vi "path steer.vi"() -> (0 "path size":i32=100, 3 "handle":dbl=-6.682613607342708)   [LabVIEW 2015]
uses:
  G_ALL.vi
panel:
  out "Array 2":dbl[][](array[numeric])
  out "dist":dbl[](array[numeric])
  in  "Numeric":dbl=2.0 format="%#_13g"
  out "Array":dbl[](array[numeric])=[0.2515789699310972, 0.252650768433432, 0.2537225783523809, 0.25479439920413827, 0.255866230504671, 0.2569380717700824, 0.25800992251627125, 0.2590817822591362, 0.2601536505146442, 0.26122552679873934, 0.2622974106272295, 0.26137675907978064, 0.26006281964444045, 0.25874890404318196, 0.2574350130090579, 0.2561211472750756, 0.25480730757403763, 0.2534934946388148, 0.2521797092019597, 0.25086595199611567, 0.24955222375374433]
  in  "y":dbl=3.0
  out "normal dist":dbl=0.8942045357809025
  out "min value":dbl=0.5
  out "size(s)":i32
  out "map_track":dbl[][](array[numeric])=[[0.15625, -20.718822434390773], [0.2395675475439587, -20.20422919806885], [0.3195188405478051, -19.689494249463262]]
  out "XY Graph":cluster{"Y":dbl[], "Y":dbl[]}[](graph)=[{"Y"=[0.15625, 0.2395675475439587, 0.3195188405478051], "Y"=[-20.718822434390773, -20.20422919806885, -19.689494249463262]}, {"Y"=array[360 elements], "Y"=array[360 elements]}, {"Y"=[0.15625, 0.2395675475439587, 0.3195188405478051], "Y"=[-20.718822434390773, -20.20422919806885, -19.689494249463262]}]
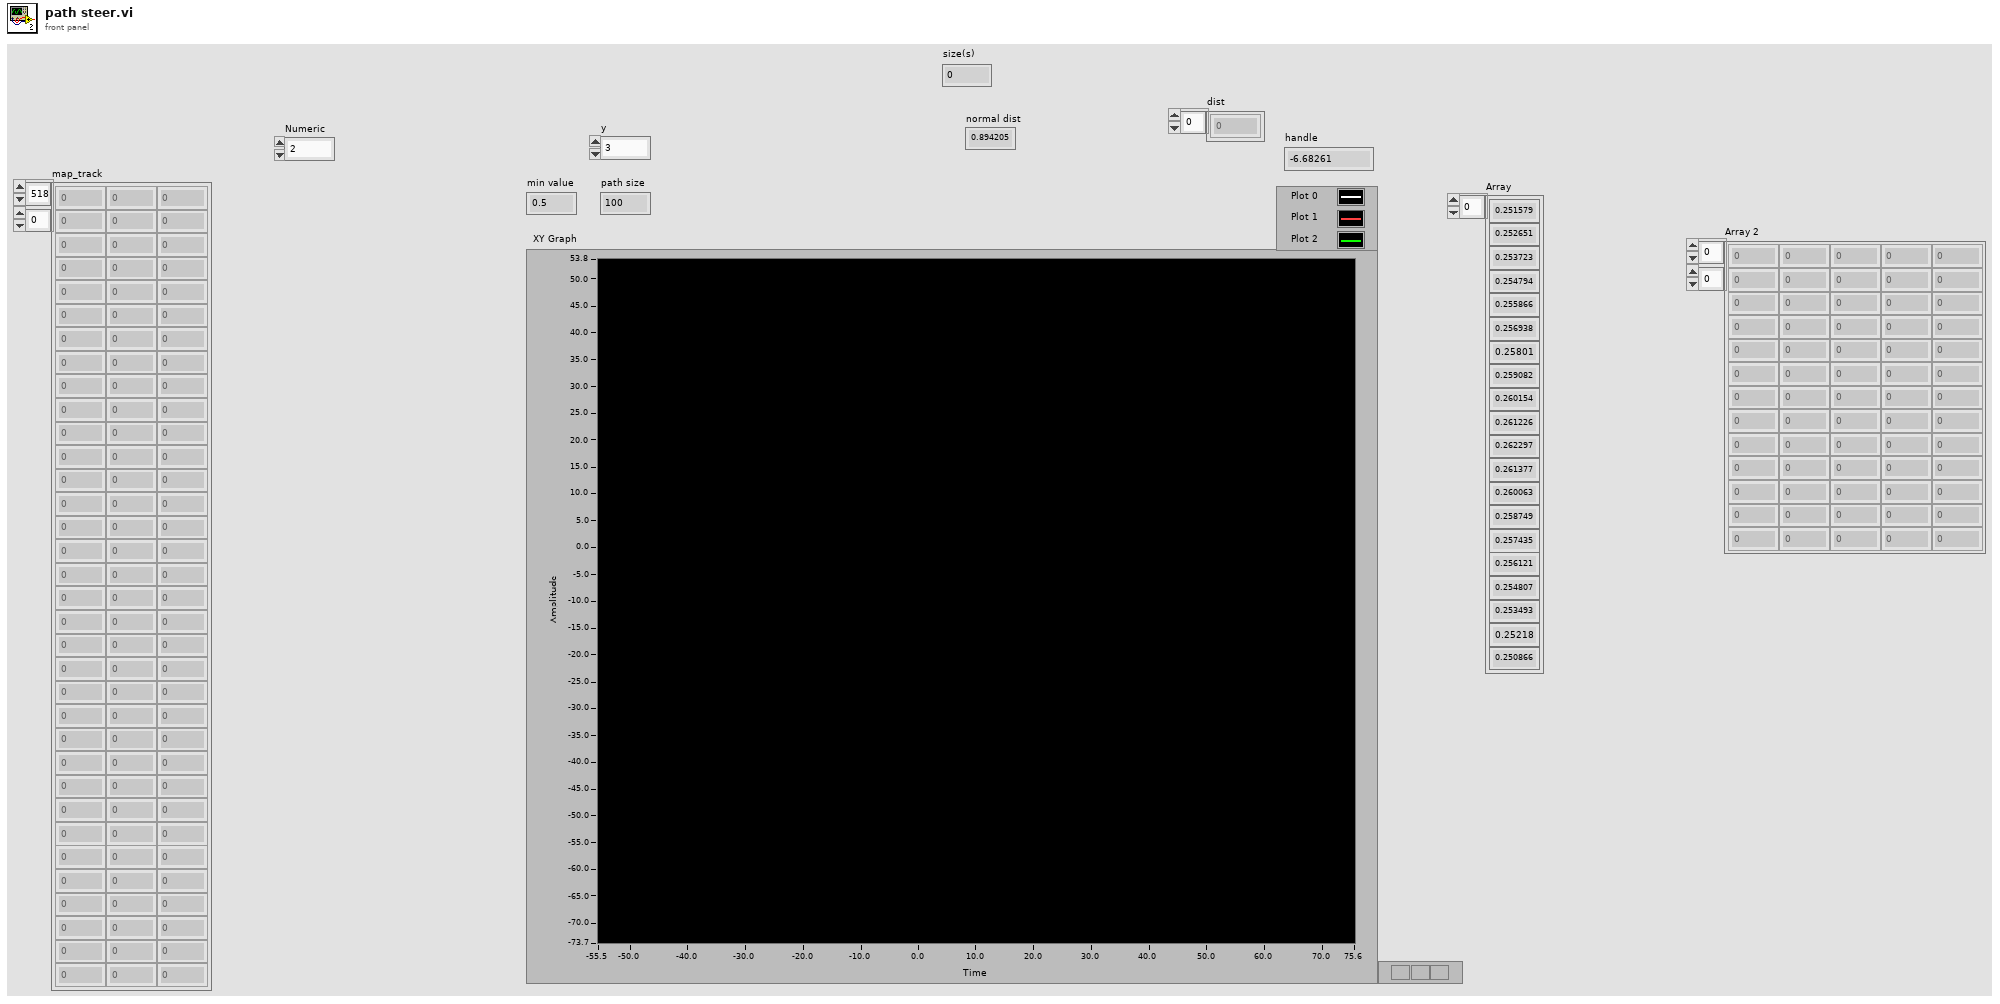
[diagram p1: front panel]
types:
  T1 = cluster{"C_Wheel base":dbl, "ratio_steer":dbl, "Overall width":dbl, "af":dbl, "turn radius":dbl, "eval":dbl, "ap":dbl, "an":dbl, "Vmax":dbl, "mu":dbl, "Vlast":dbl}
  T2 = cluster{"Steer_input":dbl, "Steer_output":dbl, "VS_des":dbl, "VS_can":dbl, "heading":dbl, "auto":bool, "run":bool, "x":dbl, "y":dbl}
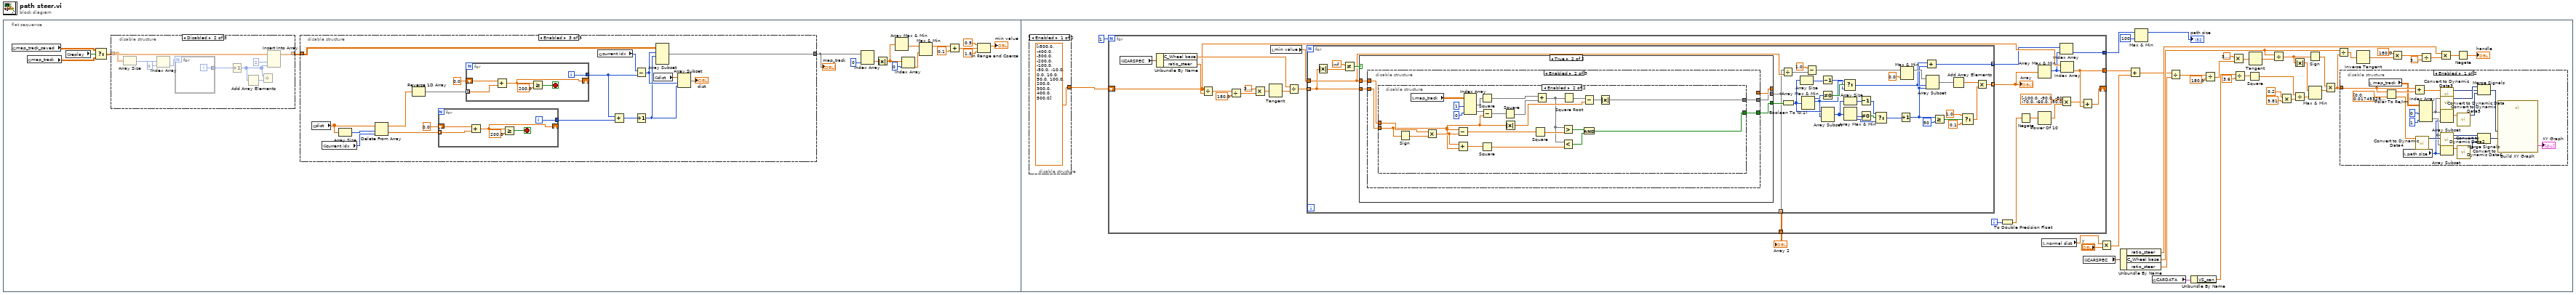
[diagram p0: block diagram]
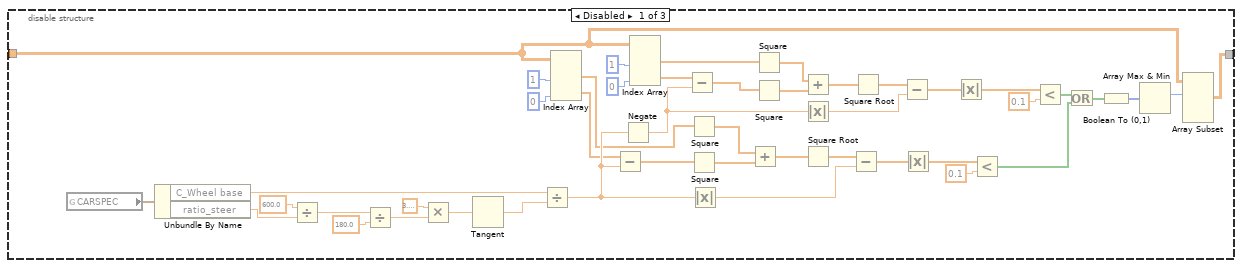
[diagram p2: hidden frame]
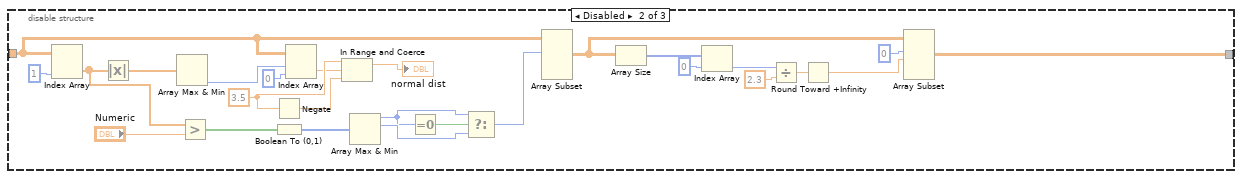
[diagram p3: hidden frame]
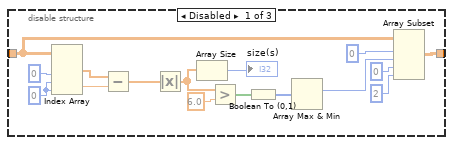
[diagram p4: hidden frame]
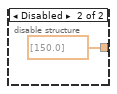
[diagram p6: hidden frame]
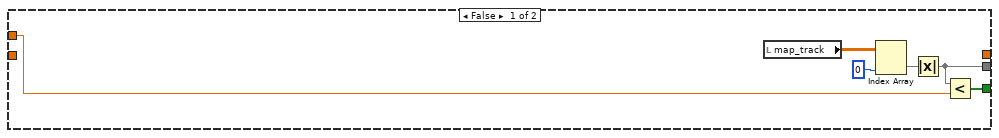
[diagram p8: hidden frame]
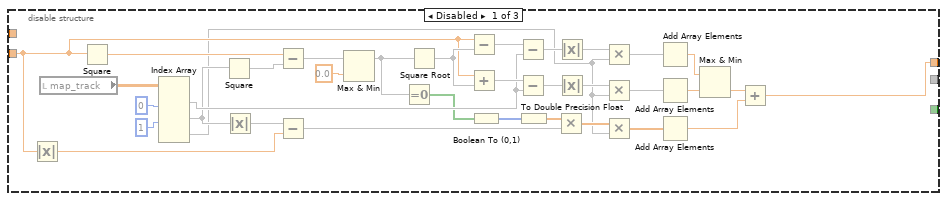
[diagram p9: hidden frame]
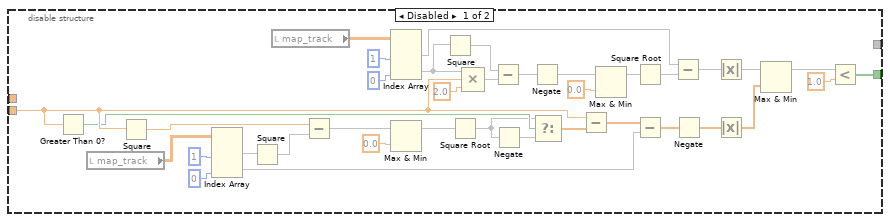
[diagram p10: hidden frame]
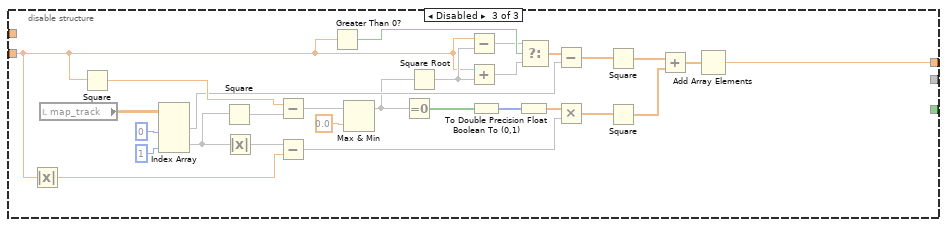
[diagram p11: hidden frame]
diagram:
  n1 = flat-sequence {
    frame #0 {
      n2 = global read "G_ALL.vi" "map_track_saved"() -> (w9:dbl[][])
      n3 = global read "G_ALL.vi" "map_track"() -> (w8:dbl[][])
      n4 = global read "G_ALL.vi" "replay"() -> (w10:bool)
      n5 = Select(t=w9, s=w10, f=w8) -> (s? t:f=w7:dbl[][])
      n6 = disable-structure shown="Disabled" {
        disable-tunnel: w7 -> [w128 w140 w146]
        disable-tunnel: [w123 w138 w146] -> w13
        frame Disabled {
          w133 = 0 ("index (col)")
          n7 = Index Array(array=w128, index (col) #1=0 ("disabled index (col)"), index (row) #2=w133, index (col) #2=w133) -> (element #1=w132:dbl[], element #2=w131:dbl)  [unwired: 1 in]
          n8 = Subtract(x=w132, y=w131) -> (x-y=w130:dbl[])
          n9 = Absolute Value(x=w130) -> (abs(x)=w122:dbl[])
          n10 = Array Size(array=w122) -> (size(s)=→"size(s)":i32)
          n11 = Greater?(x=w122, y=6.0) -> (0:w134:bool[])
          n12 = Boolean To (0,1)(Boolean=w134) -> (0, 1=w129:i16[])
          n13 = Array Max & Min(array=w129) -> (max index (indices)=w127:i32)  [unwired: 3 out]
          n14 = Array Subset(array=w128, index (row)=0 ("index"), length (row)=w127, index (col)=0 ("index"), length (col)=2 ("length")) -> (w123:dbl[][])
        }
        frame Disabled {
          n15 = Array Size(array=w140) -> (size(s)=w144:i32[])
          n16 = Index Array(array=w144, index=0) -> (element=w142:i32)
          n17 = for {
            N: w142 -> [_]
            tunnel: [w145] -> w141 mode=indexing
            i -> [w145]
          }
          n18 = Increment(x=w141) -> (x+1=w136:i32[])
          n19 = Add Array Elements(numeric array=w136) -> (sum=w137:i32)
          n20 = Divide(x=w136, y=w137) -> ()  [unwired: 1 out]
          n21 = Insert Into Array(array=w140, index (col)=2 ("disabled index (col)"), new element=w136) -> (w138:dbl[][])  [unwired: 1 in]
        }
        frame Enabled {
        }
      }
      n22 = disable-structure shown="Enabled" {
        disable-tunnel: w13 -> [w21 w74 w107]
        disable-tunnel: [w19 w87 w106] -> w11
        frame Disabled {
          n23 = global read "G_ALL.vi" "CARSPEC"() -> (w32:T1)
          n24 = Unbundle By Name(w32) -> ("C_Wheel base"=w40:dbl, "ratio_steer"=w38:dbl)
          n25 = Divide(x=600.0, y=w38) -> (x/y=w37:dbl)
          n26 = Divide(x=w37, y=180.0) -> (x/y=w34:dbl)
          n27 = Multiply(x=3.141592653589793, y=w34) -> (x*y=w36:dbl)
          n28 = Tangent(1:w36) -> (0:w39:dbl)
          n29 = Divide(x=w40, y=w39) -> (x/y=w52:dbl)
          n30 = Index Array(array=w21, index (col) #1=1 ("disabled index (col)"), index (col) #2=0 ("disabled index (col)")) -> (element #1=w27:dbl[], element #2=w29:dbl[])  [unwired: 2 in]
          n31 = Subtract(x=w29, y=w52) -> (x-y=w28:dbl[])
          n32 = Negate(x=w52) -> (-x=w53:dbl)
          n33 = Index Array(array=w21, index (col) #1=1 ("disabled index (col)"), index (col) #2=0 ("disabled index (col)")) -> (element #1=w46:dbl[], element #2=w44:dbl[])  [unwired: 2 in]
          n34 = Subtract(x=w44, y=w53) -> (x-y=w45:dbl[])
          n35 = Square(x=w27) -> (x^2=w26:dbl[])
          n36 = Square(x=w28) -> (x^2=w25:dbl[])
          n37 = Absolute Value(x=w52) -> (abs(x)=w24:dbl)
          n38 = Add(x=w26, y=w25) -> (x+y=w22:dbl[])
          n39 = Square(x=w46) -> (x^2=w47:dbl[])
          n40 = Square(x=w45) -> (x^2=w48:dbl[])
          n41 = Add(x=w47, y=w48) -> (x+y=w51:dbl[])
          n42 = Absolute Value(x=w53) -> (abs(x)=w49:dbl)
          n43 = Square Root(x=w22) -> (sqrt(x)=w23:dbl[])
          n44 = Subtract(x=w23, y=w24) -> (x-y=w60:dbl[])
          n45 = Square Root(x=w51) -> (sqrt(x)=w50:dbl[])
          n46 = Subtract(x=w50, y=w49) -> (x-y=w56:dbl[])
          n47 = Absolute Value(x=w60) -> (abs(x)=w62:dbl[])
          n48 = Absolute Value(x=w56) -> (abs(x)=w57:dbl[])
          n49 = Less?(x=w62, y=0.1) -> (x < y?=w63:bool[])
          n50 = Less?(x=w57, y=0.1) -> (x < y?=w59:bool[])
          n51 = Or(x=w59, y=w63) -> (x .or. y?=w54:bool[])
          n52 = Boolean To (0,1)(Boolean=w54) -> (0, 1=w55:i16[])
          n53 = Array Max & Min(array=w55) -> (max index (indices)=w20:i32)  [unwired: 3 out]
          n54 = Array Subset(array=w21, index (row)=w20) -> (w19:dbl[][])  [unwired: 3 in]
        }
        frame Disabled {
          w69 = 3.5 ("upper limit")
          n55 = Index Array(array=w74, index (col)=1 ("disabled index (col)")) -> (element=w76:dbl[])  [unwired: 1 in]
          n56 = Absolute Value(x=w76) -> (abs(x)=w75:dbl[])
          n57 = Array Max & Min(array=w75) -> (min index (indices)=w73:i32)  [unwired: 3 out]
          n58 = Greater?(x=w76, y="Numeric") -> (0:w83:bool[])
          n59 = Negate(x=w69) -> (-x=w70:dbl)
          n60 = Boolean To (0,1)(Boolean=w83) -> (0, 1=w82:i16[])
          n61 = Index Array(array=w74, index (row)=w73, index (col)=0 ("min index(es)")) -> (element=w68:dbl)
          n62 = In Range and Coerce(upper limit=w69, x=w68, lower limit=w70) -> (coerced(x)=→"normal dist":dbl)  [unwired: 1 out]
          n63 = Array Max & Min(array=w82) -> (max value=w79:i16, max index (indices)=w80:i32)  [unwired: 2 out]
          n64 = Equal To 0?(x=w79) -> (x = 0?=w81:bool)
          n65 = Select(t=w79, s=w81, f=w80) -> (s? t:f=w78:i32)
          n66 = Array Subset(array=w74, index (row)=w78) -> (w77:dbl[][])  [unwired: 3 in]
          n67 = Array Size(array=w77) -> (size(s)=w89:i32[])
          n68 = Index Array(array=w89, index=0) -> (element=w67:i32)
          n69 = Divide(x=w67, y=2.3) -> (x/y=w65:dbl)
          n70 = Round Toward +Infinity(x=w65) -> (ceil(x): smallest int >= x=w64:dbl)
          n71 = Array Subset(array=w77, index (row)=0 ("index"), length (row)=w64) -> (w87:dbl[][])  [unwired: 2 in]
        }
        frame Enabled {
          n72 = global read "G_ALL.vi" "dist"() -> (w104:dbl[])
          n73 = global read "G_ALL.vi" "current idx"() -> (w105:i32)
          n74 = Array Size(array=w104) -> (size(s)=w103:i32)
          n75 = Delete From Array(array=w104, length=w103, index=w105) -> (deleted portion=w99:dbl[], array with subset deleted=w102:dbl[])
          n76 = Reverse 1D Array(array=w102) -> (reversed array=w101:dbl[])
          n77 = for {
            tunnel: w99 -> [w112] mode=indexing
            shift-right: [w111] -> _
            shift-left: 0.0 -> [w113]
            tunnel: [w108] -> w95
            i -> [w108]
            stop <- w109 stop-if-true
            n78 = Add(x=w113, y=w112) -> (x+y=w111:dbl)
            n79 = Greater Or Equal?(x=w111, y=200.0) -> (x >= y?=w109:bool)
          }
          n80 = for {
            tunnel: w101 -> [w118] mode=indexing
            shift-right: [w117] -> _
            shift-left: 0.0 -> [w119]
            tunnel: [w114] -> w96
            i -> [w114]
            stop <- w115 stop-if-true
            n81 = Add(x=w119, y=w118) -> (x+y=w117:dbl)
            n82 = Greater Or Equal?(x=w117, y=200.0) -> (x >= y?=w115:bool)
          }
          n83 = global read "G_ALL.vi" "current idx"() -> (w97:i32)
          n84 = Add(x=w96, y=w95) -> (x+y=w94:i32)
          n85 = Subtract(x=w97, y=w96) -> (x-y=w92:i32)
          n86 = Increment(x=w94) -> (x+1=w91:i32)
          n87 = global read "G_ALL.vi" "dist"() -> (w93:dbl[])
          n88 = Array Subset(array=w107, index (row)=w92, length (row)=w91) -> (w106:dbl[][])  [unwired: 2 in]
          n89 = Array Subset(array=w93, index=w92, length=w91) -> (→"dist":dbl[])
        }
      }
      "map_track" <- w11
      n90 = Index Array(array=w11, index (col)=0 ("disabled index (col)")) -> (element=w6:dbl[])  [unwired: 1 in]
      n91 = Absolute Value(x=w6) -> (abs(x)=w17:dbl[])
      n92 = Array Max & Min(array=w17) -> (min value=w14:dbl)  [unwired: 3 out]
      n93 = Index Array(array=w17, index=0) -> (element=w15:dbl)
      n94 = Max & Min(x=w14, y=w15) -> (max(x,y)=w5:dbl)  [unwired: 1 out]
      n95 = Add(x=w5, y=0.1) -> (x+y=w4:dbl)
      n96 = In Range and Coerce(upper limit=0.5, x=w4, lower limit=1.5) -> (coerced(x)=→"min value":dbl)  [unwired: 1 out]
    }
    frame #1 {
      n97 = disable-structure shown="Enabled" {
        disable-tunnel: [dbl[] [-500.0, -400.0, -300.0, -200.0, -100.0, -50.0, -10.0, 0.0, 10.0, 50.0, 100.0, 200.0, 300.0, 400.0, 500.0] ("theta") dbl[] [150.0] ("theta")] -> w148
        frame Enabled {
        }
        frame Disabled {
        }
      }
      n98 = for {
        N: 1 -> [_]
        tunnel: [w221] -> w150
        shift-right: [w222] -> _
        shift-left: w148 -> [w223]
        tunnel: [w215] -> w158
        tunnel: [w214] -> w147
        i -> [w228]
        n99 = global read "G_ALL.vi" "CARSPEC"() -> (w230:T1)
        n100 = Unbundle By Name(w230) -> ("C_Wheel base"=w238:dbl, "ratio_steer"=w236:dbl)
        n101 = Divide(x=w223, y=w236) -> (x/y=w235:dbl[])
        n102 = Divide(x=w235, y=180.0) -> (x/y=w232:dbl[])
        n103 = Multiply(x=3.141592653589793, y=w232) -> (x*y=w234:dbl[])
        n104 = Tangent(1:w234) -> (0:w237:dbl[])
        n105 = local read "min value"() -> (w218:dbl)
        n106 = Divide(x=w238, y=w237) -> (x/y=w229:dbl[])
        n107 = for {
          tunnel: w229 -> [w274] mode=indexing
          tunnel: [w240] -> w219 mode=indexing
          tunnel: w218 -> [w251]
          tunnel: [w248] -> w217 mode=indexing
          tunnel: [w239] -> w214 mode=indexing
          n108 = Absolute Value(x=w274) -> (abs(x)=w272:dbl)
          n109 = Not Equal?(x=inf, y=w272) -> (x != y?=w271:bool)
          n110 = case shown="True" w271 {
            tunnel: [_ w284] -> _
            tunnel: w274 -> [_ w285]
            tunnel: [w278 w283] -> w270
            tunnel: w251 -> [w277 w282]
            tunnel: [w276 w281] -> w239
            frame False {
              n111 = local read "map_track"() -> (w275:dbl[][])
              n112 = Index Array(array=w275, index (col)=0) -> (element=w279:dbl[])  [unwired: 1 in]
              n113 = Absolute Value(x=w279) -> (abs(x)=w276:dbl[])
              n114 = Less?(x=w276, y=w277) -> (x < y?=w278:bool[])
            }
            frame True {
              n115 = disable-structure shown="Enabled" {
                disable-tunnel: w285 -> [w304 w323 w397]
                disable-tunnel: [w295 _ w399] -> w284
                disable-tunnel: [_ w322 _] -> w283
                disable-tunnel: w282 -> [_ w321 _]
                disable-tunnel: [_ w320 _] -> w281
                frame Disabled {
                  n116 = Absolute Value(x=w304) -> (abs(x)=w303:dbl)
                  n117 = local read "map_track"() -> (w293:dbl[][])
                  n118 = Square(x=w304) -> (x^2=w317:dbl)
                  n119 = Index Array(array=w293, index (col) #1=0 ("disabled index (col)"), index (col) #2=1 ("disabled index (col)")) -> (element #1=w306:dbl[], element #2=w298:dbl[], element #3=w286:dbl[])  [unwired: 4 in]
                  n120 = Square(x=w298) -> (x^2=w318:dbl[])
                  n121 = Absolute Value(x=w298) -> (abs(x)=w297:dbl[])
                  n122 = Subtract(x=w317, y=w318) -> (x-y=w309:dbl[])
                  n123 = Subtract(x=w297, y=w303) -> (x-y=w299:dbl[])
                  n124 = Max & Min(x=w309, y=0.0) -> (max(x,y)=w305:dbl[])  [unwired: 1 out]
                  n125 = Equal To 0?(x=w305) -> (x = 0?=w302:bool[])
                  n126 = Square Root(x=w305) -> (sqrt(x)=w316:dbl[])
                  n127 = Subtract(x=w304, y=w316) -> (x-y=w315:dbl[])
                  n128 = Add(x=w304, y=w316) -> (x+y=w314:dbl[])
                  n129 = Boolean To (0,1)(Boolean=w302) -> (0, 1=w301:i16[])
                  n130 = Subtract(x=w315, y=w306) -> (x-y=w313:dbl[])
                  n131 = Subtract(x=w314, y=w306) -> (x-y=w312:dbl[])
                  n132 = To Double Precision Float(number=w301) -> (double precision float=w300:dbl[])
                  n133 = Multiply(x=w300, y=w299) -> (x*y=w292:dbl[])
                  n134 = Absolute Value(x=w313) -> (abs(x)=w290:dbl[])
                  n135 = Absolute Value(x=w312) -> (abs(x)=w288:dbl[])
                  n136 = Multiply(x=w290, y=w286) -> (x*y=w289:dbl[])
                  n137 = Multiply(x=w288, y=w286) -> (x*y=w287:dbl[])
                  n138 = Multiply(x=w292, y=w286) -> (x*y=w291:dbl[])
                  n139 = Add Array Elements(numeric array=w289) -> (sum=w311:dbl)
                  n140 = Add Array Elements(numeric array=w287) -> (sum=w310:dbl)
                  n141 = Add Array Elements(numeric array=w291) -> (sum=w294:dbl)
                  n142 = Max & Min(x=w311, y=w310) -> (min(x,y)=w296:dbl)  [unwired: 1 out]
                  n143 = Add(x=w296, y=w294) -> (x+y=w295:dbl)
                }
                frame Enabled {
                  n144 = disable-structure shown="Enabled" {
                    disable-tunnel: w323 -> [w346 w366]
                    disable-tunnel: [w324 w372] -> w322
                    disable-tunnel: w321 -> [_ w367]
                    disable-tunnel: [_ w362] -> w320
                    frame Disabled {
                      n145 = Greater Than 0?(x=w346) -> (x > 0?=w345:bool)
                      n146 = local read "map_track"() -> (w350:dbl[][])
                      n147 = Square(x=w346) -> (x^2=w349:dbl)
                      n148 = Index Array(array=w350, index (col) #1=1 ("disabled index (col)"), index (col) #2=0 ("index (col)")) -> (element #1=w348:dbl[], element #2=w332:dbl[])  [unwired: 2 in]
                      n149 = Square(x=w348) -> (x^2=w347:dbl[])
                      n150 = local read "map_track"() -> (w359:dbl[][])
                      n151 = Subtract(x=w349, y=w347) -> (x-y=w337:dbl[])
                      n152 = Index Array(array=w359, index (col) #1=1 ("disabled index (col)"), index (col) #2=0 ("disabled index (col)")) -> (element #1=w353:dbl[], element #2=w357:dbl[])  [unwired: 2 in]
                      n153 = Max & Min(x=w337, y=0.0 ("value")) -> (max(x,y)=w336:dbl[])  [unwired: 1 out]
                      n154 = Square(x=w357) -> (x^2=w358:dbl[])
                      n155 = Square Root(x=w336) -> (sqrt(x)=w341:dbl[])
                      n156 = Compound Arithmetic op=MULTIPLY(w357, w346, 2.0 ("value")) -> (w355:dbl[])
                      n157 = Subtract(x=w358, y=w355) -> (x-y=w352:dbl[])
                      n158 = Negate(x=w341) -> (-x=w344:dbl[])
                      n159 = Negate(x=w352) -> (-x=w335:dbl[])
                      n160 = Select(t=w341, s=w345, f=w344) -> (s? t:f=w342:dbl[])
                      n161 = Subtract(x=w346, y=w342) -> (x-y=w334:dbl[])
                      n162 = Max & Min(x=w335, y=0.0 ("value")) -> (max(x,y)=w340:dbl[])  [unwired: 1 out]
                      n163 = Square Root(x=w340) -> (sqrt(x)=w343:dbl[])
                      n164 = Subtract(x=w334, y=w332) -> (x-y=w331:dbl[])
                      n165 = Subtract(x=w353, y=w343) -> (x-y=w330:dbl[])
                      n166 = Negate(x=w331) -> (-x=w329:dbl[])
                      n167 = Absolute Value(x=w330) -> (abs(x)=w328:dbl[])
                      n168 = Absolute Value(x=w329) -> (abs(x)=w327:dbl[])
                      n169 = Max & Min(x=w328, y=w327) -> (max(x,y)=w326:dbl[])  [unwired: 1 out]
                      n170 = Less?(x=w326, y=1.0) -> (x < y?=w324:bool[])
                    }
                    frame Enabled {
                      n171 = Sign(1:w366) -> (0:w371:dbl)
                      n172 = local read "map_track"() -> (w382:dbl[][])
                      n173 = Multiply(x=w367, y=w371) -> (x*y=w370:dbl)
                      n174 = Subtract(x=w366, y=w370) -> (x-y=w369:dbl)
                      n175 = Add(x=w370, y=w366) -> (x+y=w368:dbl)
                      n176 = Index Array(array=w382, index (col) #1=1 ("disabled index (col)"), index (col) #2=0 ("disabled index (col)")) -> (element #1=w379:dbl[], element #2=w381:dbl[])  [unwired: 2 in]
                      n177 = Square(x=w379) -> (x^2=w378:dbl[])
                      n178 = Square(x=w368) -> (x^2=w374:dbl)
                      n179 = Subtract(x=w381, y=w366) -> (x-y=w380:dbl[])
                      n180 = Square(x=w380) -> (x^2=w377:dbl[])
                      n181 = Absolute Value(x=w366) -> (abs(x)=w365:dbl)
                      n182 = Square(x=w369) -> (x^2=w376:dbl)
                      n183 = Add(x=w378, y=w377) -> (x+y=w361:dbl[])
                      n184 = Greater?(x=w361, y=w376) -> (0:w375:bool[])
                      n185 = Less?(x=w361, y=w374) -> (x < y?=w373:bool[])
                      n186 = Square Root(x=w361) -> (sqrt(x)=w364:dbl[])
                      n187 = Subtract(x=w364, y=w365) -> (x-y=w363:dbl[])
                      n188 = And(x=w375, y=w373) -> (x .and. y?=w372:bool[])
                      n189 = Absolute Value(x=w363) -> (abs(x)=w362:dbl[])
                    }
                  }
                }
                frame Disabled {
                  n190 = Absolute Value(x=w397) -> (abs(x)=w395:dbl)
                  n191 = local read "map_track"() -> (w385:dbl[][])
                  n192 = Square(x=w397) -> (x^2=w410:dbl)
                  n193 = Index Array(array=w385, index (col) #1=0 ("disabled index (col)"), index (col) #2=1 ("disabled index (col)")) -> (element #1=w405:dbl[], element #2=w398:dbl[])  [unwired: 2 in]
                  n194 = Square(x=w398) -> (x^2=w411:dbl[])
                  n195 = Absolute Value(x=w398) -> (abs(x)=w396:dbl[])
                  n196 = Subtract(x=w410, y=w411) -> (x-y=w408:dbl[])
                  n197 = Subtract(x=w396, y=w395) -> (x-y=w387:dbl[])
                  n198 = Greater Than 0?(x=w397) -> (x > 0?=w404:bool)
                  n199 = Max & Min(x=w408, y=0.0) -> (max(x,y)=w391:dbl[])  [unwired: 1 out]
                  n200 = Equal To 0?(x=w391) -> (x = 0?=w390:bool[])
                  n201 = Square Root(x=w391) -> (sqrt(x)=w409:dbl[])
                  n202 = Subtract(x=w397, y=w409) -> (x-y=w403:dbl[])
                  n203 = Add(x=w397, y=w409) -> (x+y=w401:dbl[])
                  n204 = Boolean To (0,1)(Boolean=w390) -> (0, 1=w389:i16[])
                  n205 = To Double Precision Float(number=w389) -> (double precision float=w388:dbl[])
                  n206 = Select(t=w403, s=w404, f=w401) -> (s? t:f=w402:dbl[])
                  n207 = Subtract(x=w402, y=w405) -> (x-y=w400:dbl[])
                  n208 = Multiply(x=w388, y=w387) -> (x*y=w386:dbl[])
                  n209 = Square(x=w400) -> (x^2=w394:dbl[])
                  n210 = Square(x=w386) -> (x^2=w393:dbl[])
                  n211 = Add(x=w394, y=w393) -> (x+y=w392:dbl[])
                  n212 = Add Array Elements(numeric array=w392) -> (sum=w399:dbl)
                }
              }
            }
          }
          n213 = Divide(x=w239, y=w251) -> (x/y=w252:dbl[])
          n214 = Boolean To (0,1)(Boolean=w270) -> (0, 1=w262:i16[])
          n215 = Array Size(array=w262) -> (size(s)=w261:i32)
          n216 = Array Max & Min(array=w262) -> (max value=w269:i16, max index (indices)=w259:i32)  [unwired: 2 out]
          n217 = Subtract(x=1.0, y=w252) -> (x-y=w254:dbl[])
          n218 = Decrement(x=w261) -> (x-1=w258:i32)
          n219 = Not Equal To 0?(x=w269) -> (x != 0?=w260:bool)
          n220 = Array Subset(array=w262, index=w259) -> (w267:i16[])  [unwired: 1 in]
          n221 = Select(t=w259, s=w260, f=w258) -> (s? t:f=w249:i32)
          n222 = Array Size(array=w267) -> (size(s)=w266:i32)
          n223 = Array Max & Min(array=w267) -> (min value=w268:i16, min index (indices)=w263:i32)  [unwired: 2 out]
          n224 = Decrement(x=w266) -> (x-1=w264:i32)
          n225 = Not Equal To 0?(x=w268) -> (x != 0?=w265:bool)
          n226 = Select(t=w264, s=w265, f=w263) -> (s? t:f=w257:i32)
          n227 = Increment(x=w257) -> (x+1=w247:i32)
          n228 = Max & Min(x=w254, y=0.0) -> (max(x,y)=w250:dbl[])  [unwired: 1 out]
          n229 = Add(x=w249, y=w247) -> (x+y=w248:i32)
          n230 = Array Subset(array=w250, index=w249, length=w247) -> (w256:dbl[])
          n231 = Greater Or Equal?(x=w247, y=50) -> (x >= y?=w245:bool)
          n232 = Add Array Elements(numeric array=w256) -> (sum=w242:dbl)
          n233 = Select(t=1.0, s=w245, f=0.1) -> (s? t:f=w241:dbl)
          n234 = Multiply(x=w242, y=w241) -> (x*y=w240:dbl)
        }
        "Array" <- w219
        n235 = To Double Precision Float(number=w228) -> (double precision float=w226:dbl)
        n236 = Negate(x=w226) -> (-x=w225:dbl)
        n237 = Array Max & Min(array=w219) -> (max index (indices)=w216:i32)  [unwired: 3 out]
        n238 = Power Of 10(x=w225) -> (10^x=w224:dbl)
        n239 = Index Array(array=w217, index=w216) -> (element=w215:i32)
        n240 = Multiply(x=dbl[] [-100.0, -90.0, -80.0, -70.0, -60.0, -50.0, -40.0, -30.0, -20.0, -10.0, 0.0, 10.0, 20.0, 30.0, 40.0, 50.0, 60.0, 70.0, 80.0, 90.0, 100.0], y=w224) -> (x*y=w220:dbl[])
        n241 = Index Array(array=w223, index=w216) -> (element=w221:dbl)
        n242 = Add(x=w220, y=w221) -> (x+y=w222:dbl[])
      }
      "Array 2" <- w147
      n243 = local read "normal dist"() -> (w155:dbl)
      n244 = global read "G_ALL.vi" "CARSPEC"() -> (w162:T1)
      n245 = Multiply(x=w155, y="y") -> (x*y=w153:dbl)
      n246 = Unbundle By Name(w162) -> ("ratio_steer"=w160:dbl, "C_Wheel base"=w161:dbl, "ratio_steer"=w168:dbl)
      n247 = Add(x=w150, y=w153) -> (x+y=w149:dbl)
      n248 = Max & Min(x=w158, y=100) -> (max(x,y)=→"path size":i32)  [unwired: 1 out]
      n249 = global read "G_ALL.vi" "CARDATA"() -> (w187:T2)
      n250 = Divide(x=w149, y=w168) -> (x/y=w167:dbl)
      n251 = Unbundle By Name(w187) -> ("VS_can"=w170:dbl)
      n252 = Divide(x=w167, y=180.0) -> (x/y=w164:dbl)
      n253 = Multiply(x=3.141592653589793, y=w164) -> (x*y=w166:dbl)
      n254 = Divide(x=w170, y=3.6) -> (x/y=w174:dbl)
      n255 = Square(x=w174) -> (x^2=w175:dbl)
      n256 = Tangent(1:w166) -> (0:w169:dbl)
      n257 = Divide(x=w161, y=w169) -> (x/y=w151:dbl)
      n258 = Multiply(x=0.2, y=9.81) -> (x*y=w176:dbl)
      n259 = Absolute Value(x=w151) -> (abs(x)=w177:dbl)
      n260 = Divide(x=w175, y=w176) -> (x/y=w178:dbl)
      n261 = Sign(1:w151) -> (0:w180:dbl)
      n262 = Max & Min(x=w177, y=w178) -> (max(x,y)=w179:dbl)  [unwired: 1 out]
      n263 = Multiply(x=w180, y=w179) -> (x*y=w188:dbl)
      n264 = Divide(x=w161, y=w188) -> (x/y=w186:dbl)
      n265 = disable-structure shown="Enabled" {
        disable-tunnel: w188 -> [w202 _]
        frame Enabled {
          n266 = local read "map_track"() -> (w199:dbl[][])
          n267 = Polar To Re/Im(2:dbl[] [0.0, 0.017453292519943295, 0.03490658503988659, 0.05235987755982988, 0.06981317007977318, 0.08726646259971647, 0.10471975511965977, 0.12217304763960307, 0.13962634015954636, 0.15707963267948966, 0.17453292519943295, 0.19198621771937624, 0.20943951023931953, 0.22689280275926282, 0.24434609527920614, 0.2617993877991494, 0.2792526803190927, 0.296705972839036, 0.3141592653589793, 0.33161255787892263, 0.3490658503988659, 0.3665191429188092, 0.3839724354387525, 0.40142572795869574, 0.41887902047863906, 0.4363323129985824, 0.45378560551852565, 0.47123889803846897, 0.4886921905584123, 0.5061454830783556, 0.5235987755982988, 0.5410520681182421, 0.5585053606381855, 0.5759586531581287, 0.593411945678072, 0.6108652381980153, 0.6283185307179586, 0.6457718232379019, 0.6632251157578453, 0.6806784082777886, 0.6981317007977318, 0.7155849933176751, 0.7330382858376184, 0.7504915783575618, 0.767944870877505, 0.7853981633974483, 0.8028514559173915, 0.8203047484373349, 0.8377580409572781, 0.8552113334772213, 0.8726646259971648, 0.890117918517108, 0.9075712110370513, 0.9250245035569946, 0.9424777960769379, 0.9599310885968813, 0.9773843811168246, 0.9948376736367678, 1.0122909661567112, 1.0297442586766543, 1.0471975511965976, 1.064650843716541, 1.0821041362364843, 1.0995574287564276, 1.117010721276371, 1.1344640137963142, 1.1519173063162573, 1.1693705988362009, 1.186823891356144, 1.2042771838760875, 1.2217304763960306, 1.239183768915974, 1.2566370614359172, 1.2740903539558606, 1.2915436464758039, 1.3089969389957472, 1.3264502315156905, 1.3439035240356336, 1.3613568165555772, 1.3788101090755203, 1.3962634015954636, 1.413716694115407, 1.4311699866353502, 1.4486232791552935, 1.4660765716752369, 1.48352986419518, 1.5009831567151235, 1.5184364492350666, 1.53588974175501, 1.5533430342749532, 1.5707963267948966, 1.5882496193148399, 1.605702911834783, 1.6231562043547265, 1.6406094968746698, 1.6580627893946132, 1.6755160819145563, 1.6929693744344996, 1.7104226669544427, 1.7278759594743864, 1.7453292519943295, 1.7627825445142729, 1.780235837034216, 1.7976891295541593, 1.8151424220741026, 1.8325957145940461, 1.8500490071139892, 1.8675022996339325, 1.8849555921538759, 1.902408884673819, 1.9198621771937625, 1.9373154697137058, 1.9547687622336491, 1.9722220547535922, 1.9896753472735356, 2.007128639793479, 2.0245819323134224, 2.0420352248333655, 2.0594885173533086, 2.076941809873252, 2.0943951023931953, 2.111848394913139, 2.129301687433082, 2.1467549799530254, 2.1642082724729685, 2.1816615649929116, 2.199114857512855, 2.2165681500327987, 2.234021442552742, 2.251474735072685, 2.2689280275926285, 2.2863813201125716, 2.3038346126325147, 2.321287905152458, 2.3387411976724017, 2.356194490192345, 2.373647782712288, 2.3911010752322315, 2.408554367752175, 2.426007660272118, 2.443460952792061, 2.4609142453120048, 2.478367537831948, 2.495820830351891, 2.5132741228718345, 2.530727415391778, 2.548180707911721, 2.5656340004316642, 2.5830872929516078, 2.600540585471551, 2.6179938779914944, 2.6354471705114375, 2.652900463031381, 2.670353755551324, 2.6878070480712672, 2.705260340591211, 2.7227136331111543, 2.7401669256310974, 2.7576202181510405, 2.7750735106709836, 2.792526803190927, 2.8099800957108707, 2.827433388230814, 2.844886680750757, 2.8623399732707004, 2.8797932657906435, 2.897246558310587, 2.91469985083053, 2.9321531433504737, 2.949606435870417, 2.96705972839036, 2.9845130209103035, 3.001966313430247, 3.01941960595019, 3.036872898470133, 3.0543261909900767, 3.07177948351002, 3.089232776029963, 3.1066860685499065, 3.12413936106985, 3.141592653589793, 3.159045946109736, 3.1764992386296798, 3.193952531149623, 3.211405823669566, 3.2288591161895095, 3.246312408709453, 3.2637657012293966, 3.2812189937493397, 3.2986722862692828, 3.3161255787892263, 3.3335788713091694, 3.3510321638291125, 3.368485456349056, 3.385938748868999, 3.4033920413889422, 3.4208453339088853, 3.4382986264288293, 3.455751918948773, 3.473205211468716, 3.490658503988659, 3.5081117965086026, 3.5255650890285457, 3.543018381548489, 3.560471674068432, 3.5779249665883754, 3.5953782591083185, 3.6128315516282616, 3.630284844148205, 3.647738136668149, 3.6651914291880923, 3.6826447217080354, 3.7000980142279785, 3.717551306747922, 3.735004599267865, 3.752457891787808, 3.7699111843077517, 3.787364476827695, 3.804817769347638, 3.8222710618675815, 3.839724354387525, 3.8571776469074686, 3.8746309394274117, 3.8920842319473548, 3.9095375244672983, 3.9269908169872414, 3.9444441095071845, 3.961897402027128, 3.979350694547071, 3.9968039870670142, 4.014257279586958, 4.031710572106902, 4.049163864626845, 4.066617157146788, 4.084070449666731, 4.101523742186674, 4.118977034706617, 4.136430327226561, 4.153883619746504, 4.171336912266447, 4.1887902047863905, 4.206243497306334, 4.223696789826278, 4.241150082346221, 4.258603374866164, 4.276056667386108, 4.293509959906051, 4.310963252425994, 4.328416544945937, 4.34586983746588, 4.363323129985823, 4.380776422505767, 4.39822971502571, 4.4156830075456535, 4.4331363000655974, 4.4505895925855405, 4.468042885105484, 4.485496177625427, 4.50294947014537, 4.520402762665314, 4.537856055185257, 4.5553093477052, 4.572762640225143, 4.590215932745086, 4.607669225265029, 4.625122517784973, 4.642575810304916, 4.66002910282486, 4.6774823953448035, 4.694935687864747, 4.71238898038469, 4.729842272904633, 4.747295565424576, 4.764748857944519, 4.782202150464463, 4.799655442984406, 4.81710873550435, 4.834562028024293, 4.852015320544236, 4.869468613064179, 4.886921905584122, 4.9043751981040655, 4.9218284906240095, 4.939281783143953, 4.956735075663896, 4.974188368183839, 4.991641660703782, 5.009094953223726, 5.026548245743669, 5.044001538263612, 5.061454830783556, 5.078908123303499, 5.096361415823442, 5.113814708343385, 5.1312680008633285, 5.148721293383272, 5.1661745859032155, 5.183627878423159, 5.201081170943102, 5.218534463463046, 5.235987755982989, 5.253441048502932, 5.270894341022875, 5.288347633542818, 5.305800926062762, 5.323254218582705, 5.340707511102648, 5.358160803622591, 5.3756140961425345, 5.393067388662478, 5.410520681182422, 5.427973973702365, 5.445427266222309, 5.462880558742252, 5.480333851262195, 5.497787143782138, 5.515240436302081, 5.532693728822024, 5.550147021341967, 5.567600313861911, 5.585053606381854, 5.602506898901798, 5.619960191421741, 5.6374134839416845, 5.654866776461628, 5.672320068981571, 5.689773361501514, 5.707226654021458, 5.724679946541401, 5.742133239061344, 5.759586531581287, 5.77703982410123, 5.794493116621174, 5.811946409141117, 5.82939970166106, 5.846852994181004, 5.8643062867009474, 5.8817595792208905, 5.899212871740834, 5.916666164260777, 5.93411945678072, 5.951572749300664, 5.969026041820607, 5.98647933434055, 6.003932626860494, 6.021385919380437, 6.03883921190038, 6.056292504420323, 6.073745796940266, 6.09119908946021, 6.1086523819801535, 6.126105674500097, 6.14355896702004, 6.161012259539983, 6.178465552059926, 6.19591884457987, 6.213372137099813, 6.230825429619757, 6.2482787221397, 6.265732014659643] ("x*y"), 3:w202) -> (0:w205:dbl[], 1:w201:dbl[])
          n268 = local read "path size"() -> (w194:i32)
          n269 = Add(x=w202, y=w201) -> (x+y=w200:dbl[])
          n270 = call "Convert to Dynamic Data4"("Array"=w205) -> ("Dynamic Data Type"=w204:dynamicdata)  [unwired: 3 in]
          n271 = Index Array(array=w199, index (col) #1=0 ("disabled index (col)"), index (col) #2=1 ("disabled index (col)")) -> (element #1=w198:dbl[], element #2=w195:dbl[])  [unwired: 2 in]
          n272 = call "Convert to Dynamic Data3"("Array"=w200) -> ("Dynamic Data Type"=w207:dynamicdata)  [unwired: 3 in]
          n273 = call "Convert to Dynamic Data"("Array"=w198) -> ("Dynamic Data Type"=w210:dynamicdata)  [unwired: 3 in]
          n274 = Array Subset(array=w198, length=w194) -> (w197:dbl[])  [unwired: 1 in]
          n275 = call "Convert to Dynamic Data2"("Array"=w195) -> ("Dynamic Data Type"=w209:dynamicdata)  [unwired: 3 in]
          n276 = Array Subset(array=w195, length=w194) -> (w193:dbl[])  [unwired: 1 in]
          n277 = call "Convert to Dynamic Data5"("Array"=w197) -> ("Dynamic Data Type"=w196:dynamicdata)  [unwired: 3 in]
          n278 = call "Convert to Dynamic Data6"("Array"=w193) -> ("Dynamic Data Type"=w192:dynamicdata)  [unwired: 3 in]
          n279 = Merge Signals(w210, w207, w196) -> (w208:dynamicdata)
          n280 = Merge Signals(w209, w204, w192) -> (w206:dynamicdata)
          n281 = call "Build XY Graph"("Y Input"=w206, "X Input"=w208) -> ("XY Graph"=→"XY Graph":cluster{"X":dbl[], "Y":dbl[]}[])  [unwired: 8 in, 1 out]
        }
        frame Disabled {
        }
      }
      n282 = Inverse Tangent(1:w186) -> (0:w184:dbl)
      n283 = Multiply(x=180.0 ("y"), y=w184) -> (x*y=w183:dbl)
      n284 = Divide(x=w183, y=3.141592653589793) -> (x/y=w181:dbl)
      n285 = Multiply(x=w160, y=w181) -> (x*y=w152:dbl)
      n286 = Negate(x=w152) -> (-x=→"handle":dbl)
    }
  }
